vi "Reset Statistics.vi"(8 "error in (no error)":errorcluster, 11 "L2Enet_RW_CORE in":refnum<class "L2ENET_RW_CORE.lvclass">) -> (0 "error out":errorcluster, 3 "L2Enet_RW_CORE out":refnum<class "L2ENET_RW_CORE.lvclass">)   [LabVIEW 2021, in "L2ENET_RW_CORE.lvclass"]
uses:
  L2ENET_RW_CORE.lvclass
  typedef/Statistics.ctl
  L2ENET_RW_CORE.lvclass/L2ENET_RW_CORE.ctl
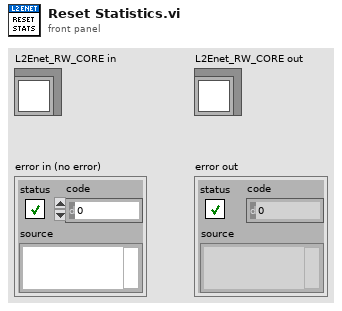
[diagram p1: front panel]
types:
  T1 = typedef "L2ENET_RW_CORE.lvclass/Statistics.ctl" = cluster{"Total Frames RW":u32, "Frames Filtered ":u32}
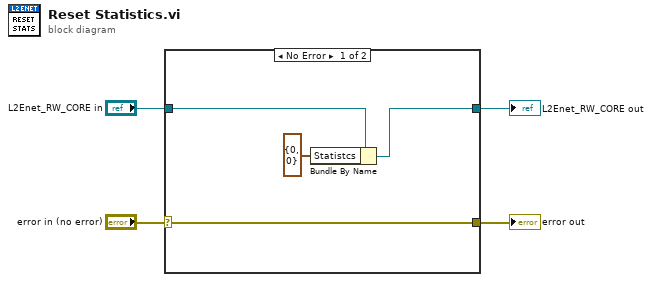
[diagram p0: block diagram]
diagram:
  n1 = case shown="No Error" "error in (no error)" {
    selector: "error in (no error)" -> [w8 w10]
    tunnel: [w8 w10] -> w3
    tunnel: [w6 w9] -> w1
    tunnel: "L2Enet_RW_CORE in" -> [w7 w9]
    frame No Error {
      n2 = Bundle By Name(cluster=w7, "Statistcs"=T1 {"Total Frames RW"=0, "Frames Filtered "=0}) -> (w6:refnum<class "L2ENET_RW_CORE.lvclass">)
    }
    frame Error {
    }
  }
  "error out" <- w3
  "L2Enet_RW_CORE out" <- w1
